vi "Exercise 2.1 – Simulated.vi"() -> ()   [LabVIEW 2024]
panel:
  out "Frequency":dbl
  out "Amplitude":dbl
  in  "stop":bool
  in  "Frequency In":dbl(knob) scale=0.0..50.0
  out "Waveform Chart":dynamicdata(graph)
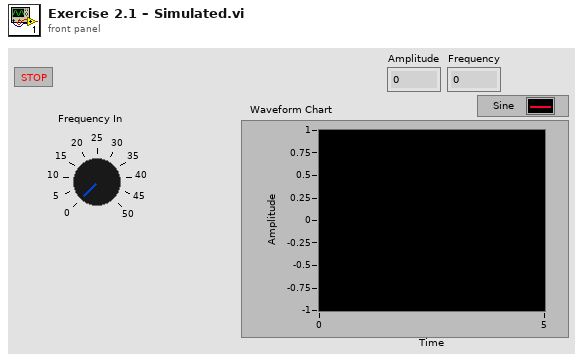
[diagram p1: front panel]
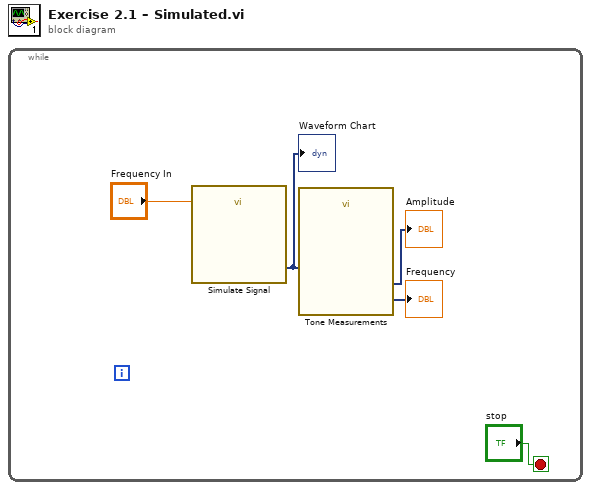
[diagram p0: block diagram]
diagram:
  n1 = while {
    stop <- "stop" stop-if-true
    n2 = call "Simulate Signal"("Frequency"="Frequency In") -> ("Sine"=w4:dynamicdata)  [unwired: 13 in, 1 out]
    "Waveform Chart" <- w4
    n3 = call "Tone Measurements"("Signals"=w4) -> ("Frequency"=→"Frequency":dynamicdata, "Amplitude"=→"Amplitude":dynamicdata)  [unwired: 8 in, 1 out]
  }
